vi "Joystick_Control_r0.vi"() -> ()   [LabVIEW 2015]
uses:
  <vilib>/Utility/inputDevices.llb/joystickAcquire.vi
  <vilib>/Utility/inputDevices.llb/closeJoystick.vi
panel:
  out "Ratioed DC":dbl
  out "Ratio B":dbl
  out "Reverse":bool
  out "Scaled Duty Cycle":dbl
  out "Ratio":dbl
  out "Right Duty Cycle":dbl
  out "Left Duty Cycle":dbl
  out "Right Turn":bool
  out "Left Turn":bool
  out "Duty Cycle":dbl
  in  "stop":bool
  out "Y axis":i32
  out "X axis":i32
  out "Dig":bool
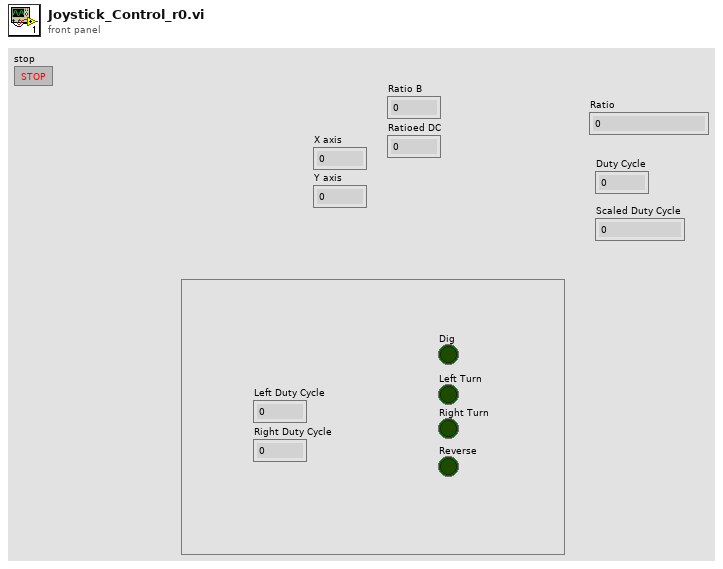
[diagram p1: front panel]
types:
  T1 = cluster{"X axis":i32, "Y axis":i32, "Z axis":i32, "X axis rotation":i32, "Y axis rotation":i32, "Z axis rotation":i32, "U axis":i32, "V axis":i32}
  T2 = cluster{"button 1":bool, "button 2":bool, "button 3":bool, "button 4":bool, "button 5":bool, "button 6":bool, "button 7":bool, "button 8":bool, "button 9":bool, "button 10":bool, "button 11":bool, "button 12":bool, "button 13":bool, "button 14":bool, "button 15":bool, "button 16":bool, "button 17":bool, "button 18":bool, "button 19":bool, "button 20":bool, "button 21":bool, "button 22":bool, "button 23":bool, "button 24":bool, "button 25":bool, "button 26":bool, "button 27":bool, "button 28":bool, "button 29":bool, "button 30":bool, "button 31":bool, "button 32":bool}
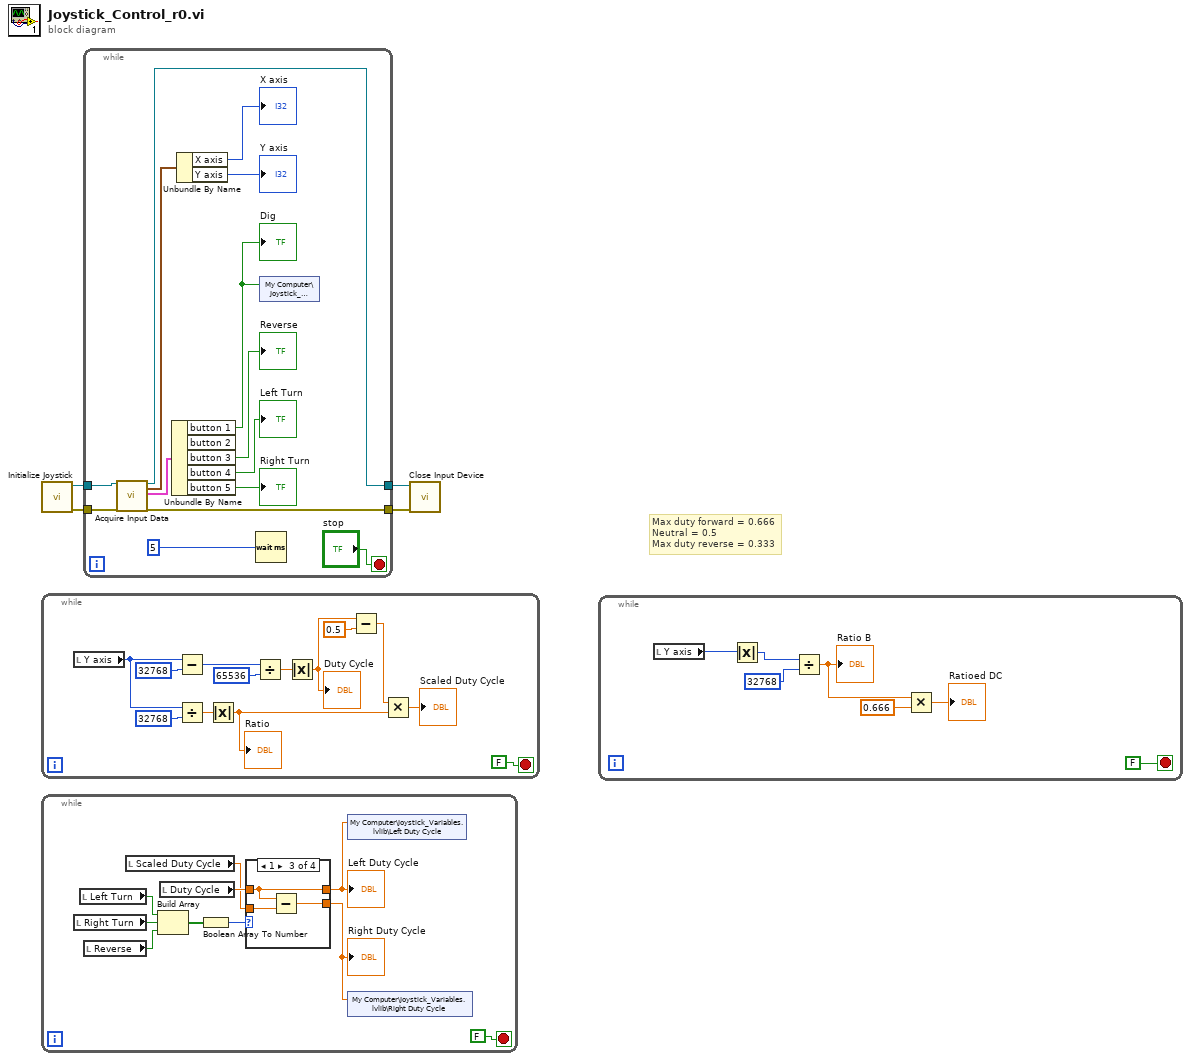
[diagram p0: block diagram]
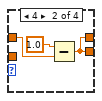
[diagram p3: hidden frame]
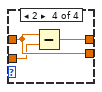
[diagram p4: hidden frame]
diagram:
  # "Max duty forward = 0.666\nNeutral = 0.5\nMax duty reverse = 0.333"
  n1 = call <vilib>:"Initialize Joystick.vi"() -> ("error out"=w2:errorcluster, "device ID"=w4:refnum<k1>)  [unwired: 10 in]
  n2 = while {
    stop <- FALSE stop-if-true
    n3 = local read "Y axis"() -> (w10:i32)
    n4 = Subtract(x=w10, y=32768) -> (x-y=w17:i32)
    n5 = Divide(x=w10, y=32768) -> (x/y=w12:dbl)
    n6 = Absolute Value(x=w12) -> (abs(x)=w9:dbl)
    "Ratio" <- w9
    n7 = Divide(x=w17, y=65536) -> (x/y=w15:dbl)
    n8 = Absolute Value(x=w15) -> (abs(x)=w7:dbl)
    "Duty Cycle" <- w7
    n9 = Subtract(x=w7, y=0.5 ("x")) -> (x-y=w5:dbl)
    n10 = Multiply(x=w5, y=w9) -> (x*y=→"Scaled Duty Cycle":dbl)
  }
  n11 = while {
    stop <- FALSE stop-if-true
    n12 = local read "Right Turn"() -> (w25:bool)
    n13 = local read "Left Turn"() -> (w26:bool)
    n14 = local read "Reverse"() -> (w20:bool)
    n15 = local read "Scaled Duty Cycle"() -> (w22:dbl)
    n16 = Build Array(w26, w25, w20) -> (w23:bool[])
    n17 = local read "Duty Cycle"() -> (w24:dbl)
    n18 = Boolean Array To Number(Boolean array=w23) -> (number=w27:u32)
    n19 = case shown="1" w27 {
      tunnel: w24 -> [w28 w30 w32 w37]
      tunnel: [w28 w29 w32 w36] -> w18
      tunnel: [w28 w29 w33 w37] -> w19
      tunnel: w22 -> [_ _ w34 w35]
      frame 0, Default {
      }
      frame 4 {
        n20 = Subtract(x=1.0, y=w30) -> (x-y=w29:dbl)
      }
      frame 1 {
        n21 = Subtract(x=w32, y=w34) -> (x-y=w33:dbl)
      }
      frame 2 {
        n22 = Subtract(x=w37, y=w35) -> (x-y=w36:dbl)
      }
    }
    "Left Duty Cycle" <- w18
    "Right Duty Cycle" <- w19
    n23 = shared-variable "My Computer\\Joystick_Variables.lvlib\\Left Duty Cycle"(w18) -> ()  [unwired: 1 in, 1 out]
    n24 = shared-variable "My Computer\\Joystick_Variables.lvlib\\Right Duty Cycle"(w19) -> ()  [unwired: 1 in, 1 out]
  }
  n25 = while {
    tunnel: w4 -> [w51]
    tunnel: [w50] -> w3
    tunnel: w2 -> [w49]
    tunnel: [w48] -> w1
    stop <- "stop" stop-if-true
    n26 = call-poly <vilib>:"Acquire Input Data.vi"("device ID"=w51, "error in (no error)"=w49) -> ("device ID"=w50:refnum<k1>, "axis info"=w47:T1, "button info"=w46:T2, "error out"=w48:errorcluster)  [unwired: 13 in, 1 out]
    n27 = Unbundle By Name(w46) -> ("button 1"=w39:bool, "button 3"=→"Reverse":bool, "button 4"=→"Left Turn":bool, "button 5"=→"Right Turn":bool)  [unwired: 1 out]
    "Dig" <- w39
    n28 = Unbundle By Name(w47) -> ("X axis"=→"X axis":i32, "Y axis"=→"Y axis":i32)
    n29 = Wait (ms)(milliseconds to wait=u32 5) -> ()  [unwired: 1 out]
    n30 = shared-variable "My Computer\\Joystick_Variables.lvlib\\Dig"(w39) -> ()  [unwired: 1 in, 1 out]
  }
  n31 = call-poly <vilib>:"Close Input Device.vi"("error in (no error)"=w1, "device ID"=w3) -> ()  [unwired: 8 in, 1 out]
  n32 = while {
    stop <- FALSE stop-if-true
    n33 = local read "Y axis"() -> (w58:i32)
    n34 = Absolute Value(x=w58) -> (abs(x)=w57:i32)
    n35 = Divide(x=w57, y=32768) -> (x/y=w55:dbl)
    "Ratio B" <- w55
    n36 = Multiply(x=w55, y=0.666) -> (x*y=→"Ratioed DC":dbl)
  }
